vi "SaveVector.vi"(8 "error in (no error)":errorcluster, 11 "Vector Refnum":refnum<k24>) -> (0 "error out":errorcluster, 3 "LEAPvector":T1)   [LabVIEW 2017, in "LeapMotion.lvlib"]
uses:
  LeapMotion.lvlib
  TypeDefs/LEAPvector.ctl
  C:/Users/snordinh/Desktop/LEAP/LEAP-sign-language-test/LeapMotion/Dynamic Libraries/LeapCSharp.NET4.5.dll
  Dynamic Libraries/LeapCSharp.NET4.5.dll
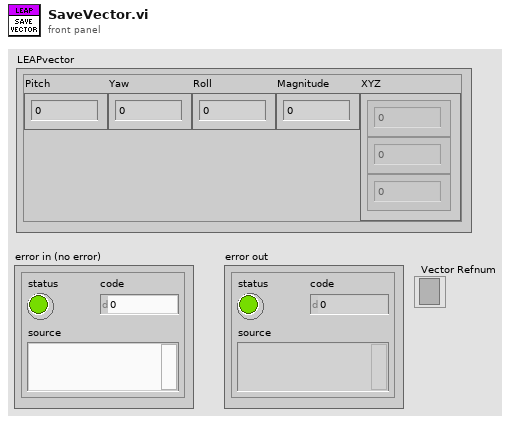
[diagram p1: front panel]
types:
  T1 = typedef "LeapMotion.lvlib/LEAPvector.ctl" = cluster{"Pitch":sgl, "Yaw":sgl, "Roll":sgl, "Magnitude":sgl, "XYZ":sgl[]}
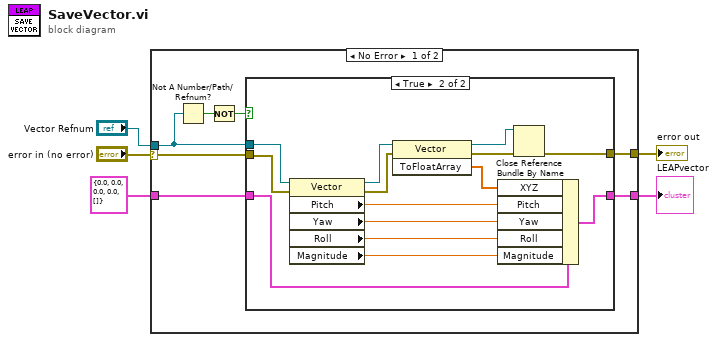
[diagram p0: block diagram]
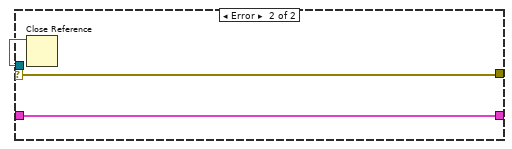
[diagram p3: hidden frame]
diagram:
  n1 = case shown="No Error" "error in (no error)" {
    selector: "error in (no error)" -> [w10 w30]
    tunnel: "Vector Refnum" -> [w9 w31]
    tunnel: T1 {"Pitch"=0.0, "Yaw"=0.0, "Roll"=0.0, "Magnitude"=0.0, "XYZ"=[]} ("LEAPvector") -> [w8 w29]
    tunnel: [w7 w30] -> w4
    tunnel: [w6 w29] -> w5
    frame No Error {
      n2 = Not A Number/Path/Refnum?(number/path/refnum=w9) -> (NaN/Path/Refnum?=w11:bool)
      n3 = Not(x=w11) -> (.not. x?=w12:bool)
      n4 = case shown="True" w12 {
        tunnel: w10 -> [w13 w27]
        tunnel: w9 -> [_ w28]
        tunnel: w8 -> [w14 w15]
        tunnel: [w13 w17] -> w7
        tunnel: [w14 w16] -> w6
        frame False {
        }
        frame True {
          n5 = property class="Vector"(reference=w28, error in=w27) -> (reference out=w22:refnum<k24>, error out=w21:errorcluster, "Pitch"=w26:sgl, "Yaw"=w25:sgl, "Roll"=w24:sgl, "Magnitude"=w23:sgl)
          n6 = invoke class="Vector" method="ToFloatArray"(reference=w22, error in=w21) -> (reference out=w18:refnum<k24>, error out=w19:errorcluster, "ToFloatArray"=w20:sgl[])  [unwired: 1 in]
          n7 = Bundle By Name(cluster=w15, "XYZ"=w20, "Pitch"=w26, "Yaw"=w25, "Roll"=w24, "Magnitude"=w23) -> (w16:T1)
          n8 = Close Reference(reference=w18, error in (no error)=w19) -> (error out=w17:errorcluster)
        }
      }
    }
    frame Error {
      n9 = Close Reference(reference=w31) -> ()  [unwired: 1 in, 1 out]
    }
  }
  "LEAPvector" <- w5
  "error out" <- w4
